vi "marker on trace.vi"() -> ()   [LabVIEW 2016]
panel:
  out "subarray 3":dbl[](array[numeric])
  out "subarray 4":dbl[](array[numeric])
  out "subarray 5":dbl[](array[numeric])
  out "subarray 2":dbl[](array[numeric])
  out "subarray 1":dbl[](array[numeric])
  out "subarray 0":dbl[](array[numeric])
  out "sorted array":dbl[][](array[numeric])
  in  "Column to Sort on":i32=1
  out "appended array":dbl[][](array[numeric])
  out "x-y":dbl[](array[numeric])
  out "limit":dbl[](array[numeric])
  out "XY Graph":cluster{i32[], dbl[]}[](graph)
  out "value":dbl[](array[numeric])
  out "X-axis":dbl[](array[numeric])
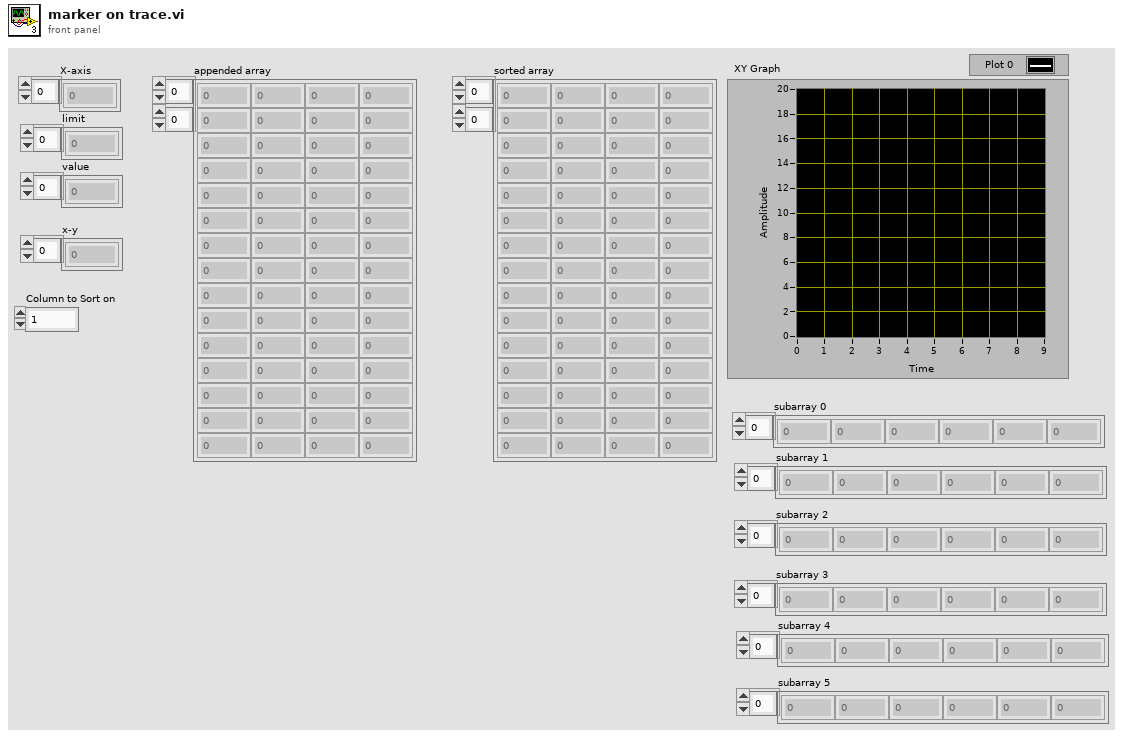
[diagram p1: front panel]
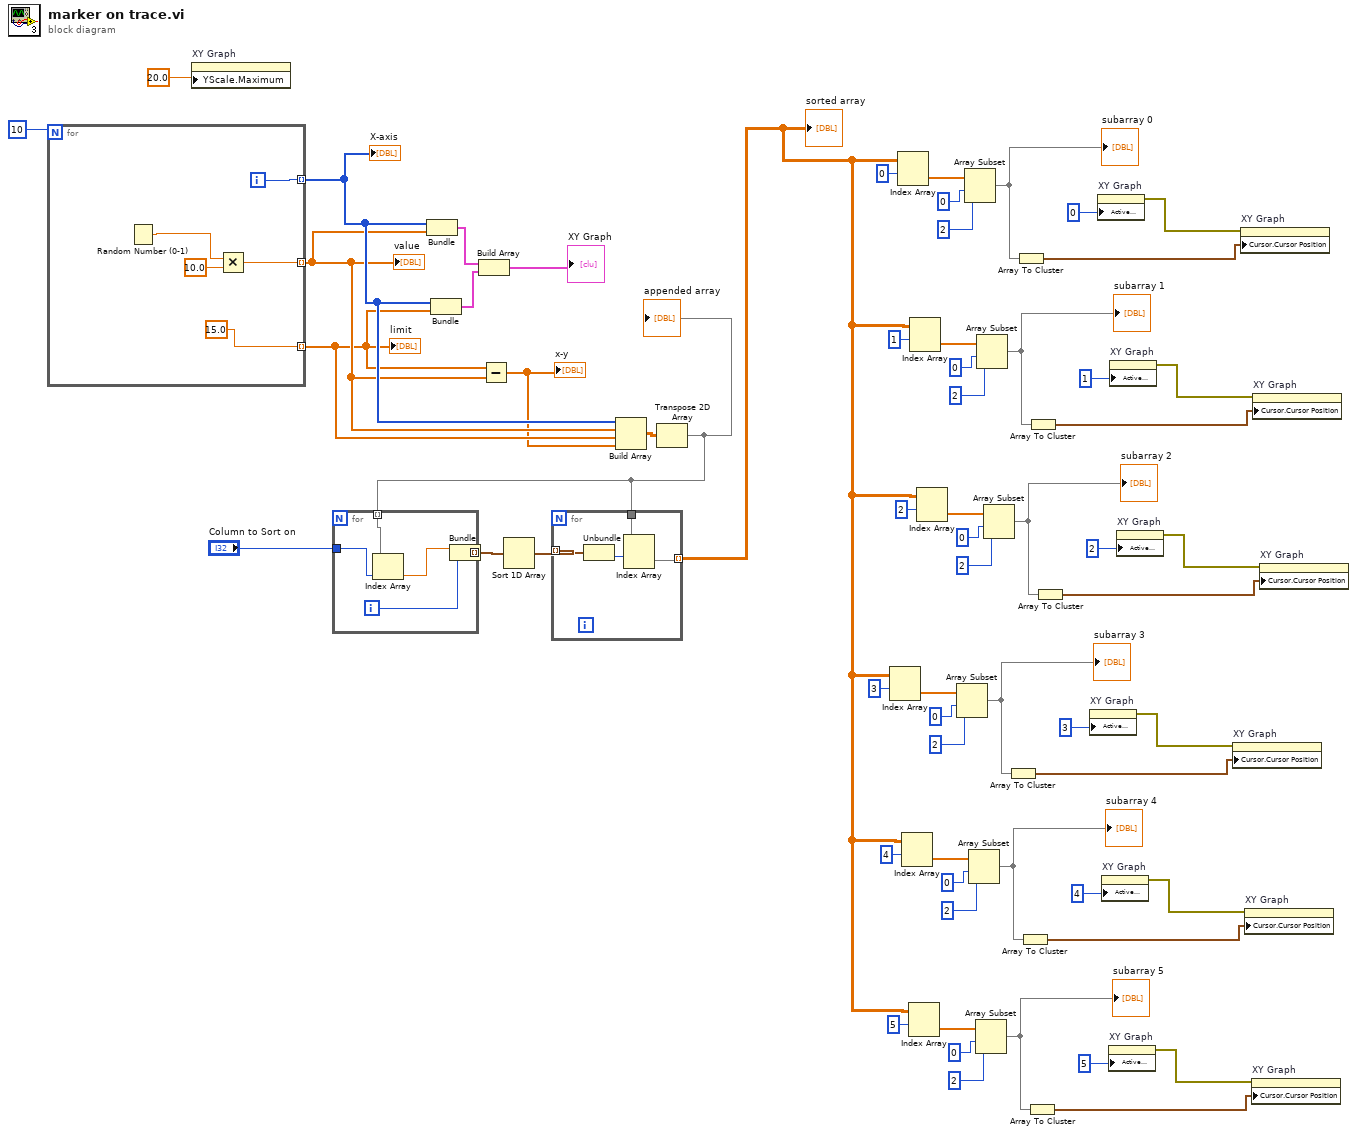
[diagram p0: block diagram]
diagram:
  n1 = for {
    N: 10 -> [_]
    tunnel: [w65] -> w58 mode=indexing
    tunnel: [w66] -> w57 mode=indexing
    tunnel: [15.0] -> w56 mode=indexing
    i -> [w65]
    n2 = Random Number (0-1)() -> (number: 0 to 1=w67:dbl)
    n3 = Multiply(x=w67, y=10.0) -> (x*y=w66:dbl)
  }
  "X-axis" <- w58
  "value" <- w57
  "limit" <- w56
  n4 = property on="XY Graph" class="XYGraph (strict)"("YScale.Maximum"=20.0 ("Y Scale.Range:Maximum")) -> ()  [unwired: 2 in, 2 out]
  n5 = Bundle(w58, w57) -> (w62:cluster{i32[], dbl[]})  [unwired: 1 in]
  n6 = Bundle(w58, w56) -> (w61:cluster{i32[], dbl[]})  [unwired: 1 in]
  n7 = Build Array(w62, w61) -> (→"XY Graph":cluster{i32[], dbl[]}[])
  n8 = Subtract(x=w56, y=w57) -> (x-y=w55:dbl[])
  "x-y" <- w55
  n9 = Build Array(w58, w57, w56, w55) -> (w51:dbl[][])
  n10 = Transpose 2D Array(2D array=w51) -> (transposed array=w50:dbl[][])
  "appended array" <- w50
  n11 = for {
    tunnel: w50 -> [w69] mode=indexing
    tunnel: [w71] -> w53 mode=indexing
    tunnel: "Column to Sort on" -> [w73]
    i -> [w72]
    n12 = Index Array(array=w69, index=w73) -> (element=w70:dbl)
    n13 = Bundle(w70, w72) -> (w71:cluster{dbl, i32})  [unwired: 1 in]
  }
  n14 = Sort 1D Array(array=w53) -> (sorted array=w52:cluster{dbl, i32}[])
  n15 = for {
    tunnel: w52 -> [w77] mode=indexing
    tunnel: [w75] -> w1 mode=indexing
    tunnel: w50 -> [w76]
    n16 = Unbundle(w77) -> (w74:i32)  [unwired: 1 out]
    n17 = Index Array(array=w76, index (row)=w74) -> (element=w75:dbl[])  [unwired: 1 in]
  }
  "sorted array" <- w1
  n18 = Index Array(array=w1, index (row)=3) -> (element=w5:dbl[])  [unwired: 1 in]
  n19 = Index Array(array=w1, index (row)=0) -> (element=w46:dbl[])  [unwired: 1 in]
  n20 = Index Array(array=w1, index (row)=4) -> (element=w14:dbl[])  [unwired: 1 in]
  n21 = Index Array(array=w1, index (row)=5) -> (element=w21:dbl[])  [unwired: 1 in]
  n22 = Index Array(array=w1, index (row)=1) -> (element=w37:dbl[])  [unwired: 1 in]
  n23 = Index Array(array=w1, index (row)=2) -> (element=w30:dbl[])  [unwired: 1 in]
  n24 = Array Subset(array=w5, index=0, length=2) -> (w8:dbl[])
  "subarray 3" <- w8
  n25 = Array Subset(array=w46, index=0, length=2) -> (w43:dbl[])
  "subarray 0" <- w43
  n26 = Array Subset(array=w14, index=0, length=2) -> (w11:dbl[])
  "subarray 4" <- w11
  n27 = Array Subset(array=w21, index=0, length=2) -> (w24:dbl[])
  "subarray 5" <- w24
  n28 = Array Subset(array=w37, index=0, length=2) -> (w40:dbl[])
  "subarray 1" <- w40
  n29 = Array Subset(array=w30, index=0, length=2) -> (w27:dbl[])
  "subarray 2" <- w27
  n30 = Array To Cluster(array=w8) -> (cluster=w9:cluster{"[0]":dbl, "[1]":dbl})
  n31 = Array To Cluster(array=w43) -> (cluster=w42:cluster{"[0]":dbl, "[1]":dbl})
  n32 = Array To Cluster(array=w11) -> (cluster=w10:cluster{"[0]":dbl, "[1]":dbl})
  n33 = Array To Cluster(array=w24) -> (cluster=w25:cluster{"[0]":dbl, "[1]":dbl})
  n34 = Array To Cluster(array=w40) -> (cluster=w41:cluster{"[0]":dbl, "[1]":dbl})
  n35 = Array To Cluster(array=w27) -> (cluster=w26:cluster{"[0]":dbl, "[1]":dbl})
  n36 = property on="XY Graph" class="XYGraph (strict)"("Active Cursor"=u32 3) -> (error out=w2:errorcluster)  [unwired: 2 in, 1 out]
  n37 = property on="XY Graph" class="XYGraph (strict)"("Active Cursor"=u32 0) -> (error out=w49:errorcluster)  [unwired: 2 in, 1 out]
  n38 = property on="XY Graph" class="XYGraph (strict)"("Active Cursor"=u32 4) -> (error out=w17:errorcluster)  [unwired: 2 in, 1 out]
  n39 = property on="XY Graph" class="XYGraph (strict)"("Active Cursor"=u32 5) -> (error out=w18:errorcluster)  [unwired: 2 in, 1 out]
  n40 = property on="XY Graph" class="XYGraph (strict)"("Active Cursor"=u32 1) -> (error out=w34:errorcluster)  [unwired: 2 in, 1 out]
  n41 = property on="XY Graph" class="XYGraph (strict)"("Active Cursor"=u32 2) -> (error out=w33:errorcluster)  [unwired: 2 in, 1 out]
  n42 = property on="XY Graph" class="XYGraph (strict)"(error in=w2, "Cursor.Cursor Position"=w9) -> ()  [unwired: 1 in, 2 out]
  n43 = property on="XY Graph" class="XYGraph (strict)"(error in=w49, "Cursor.Cursor Position"=w42) -> ()  [unwired: 1 in, 2 out]
  n44 = property on="XY Graph" class="XYGraph (strict)"(error in=w17, "Cursor.Cursor Position"=w10) -> ()  [unwired: 1 in, 2 out]
  n45 = property on="XY Graph" class="XYGraph (strict)"(error in=w18, "Cursor.Cursor Position"=w25) -> ()  [unwired: 1 in, 2 out]
  n46 = property on="XY Graph" class="XYGraph (strict)"(error in=w34, "Cursor.Cursor Position"=w41) -> ()  [unwired: 1 in, 2 out]
  n47 = property on="XY Graph" class="XYGraph (strict)"(error in=w33, "Cursor.Cursor Position"=w26) -> ()  [unwired: 1 in, 2 out]
